vi "Match ROM.vi"(7 "1-Wire DIO Pin":refnum<k21>="ConnectorA/DIO15", 8 "error in (no error)":errorcluster, 10 "ROM Code":u64) -> (0 "error out":errorcluster)   [LabVIEW 2014, in "Maxim 1-Wire.lvlib"]
doc: "MATCH ROM [55h]\nThe match ROM command followed by a 64-bit ROM code sequence allows the bus master to address a specific slave device on a multidrop or single-drop bus. Only the slave that exactly matches the 64-bit ROM code sequence will respond to the function command issued by the master; all other slaves on the bus will wait for a reset pulse."
uses:
  Maxim 1-Wire.lvlib
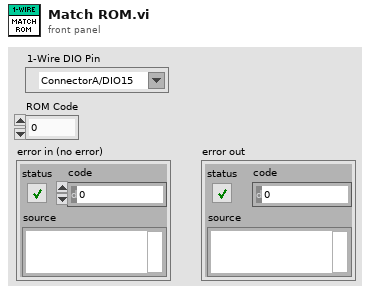
[diagram p1: front panel]
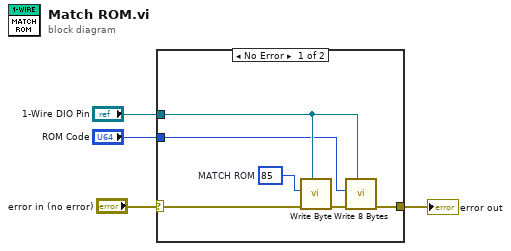
[diagram p0: block diagram]
diagram:
  n1 = case shown="No Error" "error in (no error)" {
    selector: "error in (no error)" -> [w9 w11]
    tunnel: [w7 w11] -> w4
    tunnel: "1-Wire DIO Pin" -> [w6 _]
    tunnel: "ROM Code" -> [w5 _]
    frame No Error {
      w10 = u8 85  # MATCH ROM
      n2 = call "Write Byte.vi"("1-Wire DIO Pin"=w6, "error in"=w9, "Tx data"=w10) -> ("error out"=w8:errorcluster)  [unwired: 8 in]
      n3 = call "Write 8 Bytes.vi"("1-Wire DIO Pin"=w6, "error in"=w8, "Tx data"=w5) -> ("error out"=w7:errorcluster)  [unwired: 8 in]
    }
    frame Error {
    }
  }
  "error out" <- w4
